vi "Set Image Array Size.vi"(10 "Buttons Displayed":i32, 11 "Button Images in":T1[](array[typedef])) -> (3 "Button Images out":T1[](array[typedef]))   [LabVIEW 2012, in "Button.lvclass"]
doc: "Force the image data array to be a fixed minimum size"
uses:
  Button.lvclass
  <vilib>/picture/picture.llb/imagedata.ctl
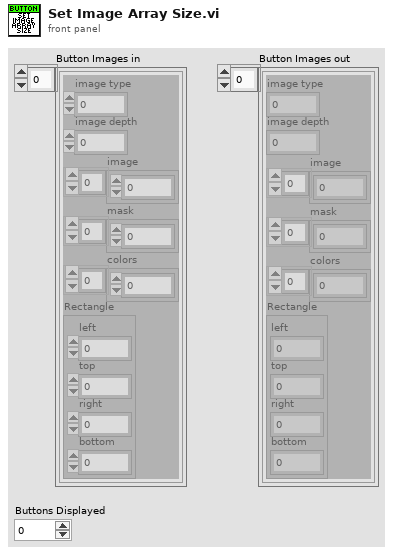
[diagram p1: front panel]
types:
  T1 = typedef "imagedata.ctl" = cluster{"image type":i32, "image depth":i32, "image":u8[], "mask":u8[], "colors":u32[], "Rectangle":cluster{"left":i16, "top":i16, "right":i16, "bottom":i16}}
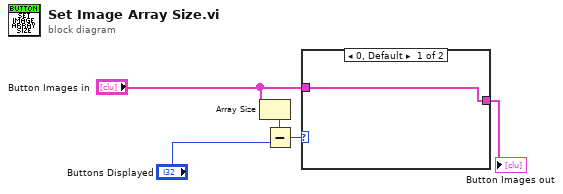
[diagram p0: block diagram]
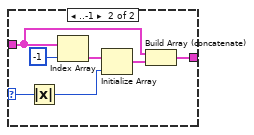
[diagram p2: hidden frame]
diagram:
  n1 = Array Size(array="Button Images in") -> (size(s)=w1:i32)
  n2 = Subtract(x=w1, y="Buttons Displayed") -> (x-y=w3:i32)
  n3 = case shown="0, Default" w3 {
    selector: w3 -> [_ w13]
    tunnel: "Button Images in" -> [w6 w10]
    tunnel: [w6 w7] -> w5
    frame 0, Default {
    }
    frame ..-1 {
      n4 = Absolute Value(x=w13) -> (abs(x)=w11:i32)
      n5 = Index Array(array=w10, index=-1) -> (element=w8:T1)
      n6 = Initialize Array(w8, w11) -> (w12:T1[])
      n7 = Build Array (concatenate)(w10, w12) -> (w7:T1[])
    }
  }
  "Button Images out" <- w5
